vi "reward_behavior_michelle_visjitter_conswinAdapt_enticefx_TSLog_VF_fortraining_lightdetection.vi"() -> ()   [LabVIEW 2019]
doc: "The myRIO Project template acquires acceleration data from the onboard accelerometer and displays the changes of acceleration values in a waveform chart."
uses:
  <vilib>/Analysis/Matrix/Datatypes/RealMatrix.ctl
  <vilib>/myRIO/Instrument Drivers/Onboard IO/DIO/typedefs/DIO Reference.ctl
  <vilib>/myRIO/Common/Instrument Driver Framework/Utilities/typedefs/myRIO Generic Hardware Reference.ctl
  <vilib>/myRIO/Common/Instrument Driver Framework/Utilities/typedefs/Hardware Version Enum.ctl
  <vilib>/myRIO/Common/Instrument Driver Framework/Utilities/typedefs/myRIO v1.0 Reference.ctl
  <vilib>/myRIO/Common/Instrument Driver Framework/Utilities/typedefs/Generic FPGA Reference.ctl
  <vilib>/myRIO/Common/Instrument Driver Framework/myRIO v1.0/DIO/typedefs/DIO Channels List.ctl
  <vilib>/myRIO/Common/Instrument Driver Framework/myRIO v1.0/DIO/typedefs/DIO Channels Enum.ctl
  <vilib>/userdefined/High Color/nirio_resource_hc.ctl
  <vilib>/myRIO/Common/Instrument Driver Framework/myRIO v1.0/Encoder/typedefs/Encoder Signal Mode.ctl
  <vilib>/myRIO/Instrument Drivers/Onboard IO/Encoder/typedefs/Encoder Reference.ctl
  <vilib>/myRIO/Common/Instrument Driver Framework/myRIO v1.0/Encoder/typedefs/Encoder Channels Enum.ctl
  <vilib>/myRIO/Common/Instrument Driver Framework/myRIO v1.0/Encoder/typedefs/Encoder Configuration v1.0.ctl
  <vilib>/myRIO/Instrument Drivers/Onboard IO/AI/typedefs/AI Reference.ctl
  <vilib>/myRIO/Common/Instrument Driver Framework/myRIO v1.0/AI/typedefs/AI Channels List.ctl
  <vilib>/myRIO/Common/Instrument Driver Framework/myRIO v1.0/AI/typedefs/AI Channels Enum.ctl
  <vilib>/myRIO/Common/Instrument Driver Framework/Utilities/typedefs/Analog Scaling Constants List.ctl
  <vilib>/myRIO/Common/Instrument Driver Framework/Utilities/typedefs/Analog Scaling Constants.ctl
  <vilib>/myRIO/Common/Instrument Driver Framework/Utilities/vis/Is FPGA Ref Available.vi
  <vilib>/myRIO/Common/Instrument Driver Framework/myRIO v1.0/DIO/vis/myRIO v1.1 Open DIO.vi
  <vilib>/myRIO/Instrument Drivers/Onboard IO/DIO/vis/Write.vi
  <vilib>/myRIO/Common/Instrument Driver Framework/myRIO v1.0/Encoder/vis/myRIO v1.1 Open Encoder.vi
  <vilib>/myRIO/Instrument Drivers/Onboard IO/Encoder/vis/Read.vi
  <vilib>/myRIO/Common/Instrument Driver Framework/myRIO v1.0/AI/vis/myRIO v1.1 Open AI.vi
  <vilib>/myRIO/Instrument Drivers/Onboard IO/AI/vis/Read.vi
  <vilib>/myRIO/Instrument Drivers/Onboard IO/DIO/vis/Read.vi
  <vilib>/myRIO/Common/Instrument Driver Framework/Utilities/vis/Validate Channels.vi
  <vilib>/myRIO/Common/Instrument Driver Framework/myRIO v1.0/DIO/vis/myRIO v1.0 Reserve DIO.vi
  <vilib>/myRIO/Common/Instrument Driver Framework/myRIO v1.0/Encoder/vis/myRIO v1.0 Reserve Encoder.vi
  <vilib>/myRIO/Common/Instrument Driver Framework/myRIO v1.0/AI/vis/myRIO v1.0 Reserve AI.vi
  <vilib>/myRIO/Common/Instrument Driver Framework/myRIO v1.0/Resource Manager/vis/myRIO v1.0 Reserve Channel List.vi
  <vilib>/myRIO/Common/Instrument Driver Framework/myRIO v1.0/DIO/vis/myRIO v1.0 Build MUX Configuration DIO.vi
  <vilib>/myRIO/Common/Instrument Driver Framework/myRIO v1.0/Encoder/vis/myRIO v1.0 Build MUX Configuration Encoder.vi
  <vilib>/myRIO/Common/Instrument Driver Framework/myRIO v1.0/AI/vis/myRIO v1.0 Build MUX Configuration AI.vi
  <vilib>/myRIO/Common/Instrument Driver Framework/myRIO v1.0/Resource Manager/vis/myRIO v1.0 Reserve Channel.vi
  <vilib>/myRIO/Common/Instrument Driver Framework/myRIO v1.0/Resource Manager/vis/myRIO v1.0 Unreserve Channel.vi
  <vilib>/myRIO/Common/Instrument Driver Framework/myRIO v1.0/Resource Manager/vis/myRIO v1.0 Create Configuration List.vi
  <vilib>/myRIO/Common/Instrument Driver Framework/myRIO v1.0/Resource Manager/vis/myRIO v1.0 Build Mutex Name.vi
  <vilib>/Utility/VariantDataType/GetNumericInfo.vi
  <vilib>/Utility/error.llb/Error Cluster From Error Code.vi
  <vilib>/myRIO/Common/Instrument Driver Framework/myRIO v1.0/myRIO v1.1 Open.vi
  <vilib>/myRIO/Common/Instrument Driver Framework/Utilities/vis/IO Manager.vi
  <vilib>/myRIO/Common/Instrument Driver Framework/Utilities/vis/Configuration Manager.vi
  <vilib>/myRIO/Common/Instrument Driver Framework/myRIO v1.0/Resource Manager/vis/myRIO v1.0 Configure IO.vi
  <vilib>/myRIO/Common/Instrument Driver Framework/myRIO v1.0/myRIO v1.0 Close.vi
  <vilib>/myRIO/Common/Instrument Driver Framework/myRIO v1.0/Encoder/vis/myRIO v1.0 Configure Encoder.vi
  <vilib>/myRIO/Common/Instrument Driver Framework/myRIO v1.0/Encoder/vis/myRIO v1.0 Read Encoder.vi
  <vilib>/myRIO/Common/Instrument Driver Framework/myRIO v1.0/DIO/vis/myRIO v1.0 Write DIO.vi
  <vilib>/myRIO/Common/Instrument Driver Framework/myRIO v1.0/DIO/vis/myRIO v1.0 Read DIO.vi
  <vilib>/myRIO/Common/Instrument Driver Framework/myRIO v1.0/AI/vis/myRIO v1.0 Get Scaling Constants AI.vi
  <vilib>/myRIO/Common/Instrument Driver Framework/myRIO v1.0/AI/vis/myRIO v1.0 Read AI.vi
  <vilib>/myRIO/Express VI/Onboard IO/Encoder/Encoder Express VI.xnode
  <vilib>/myRIO/Instrument Drivers/Onboard IO/Encoder/vis/myRIO Encoder Open.xnode
  <vilib>/myRIO/Common/Instrument Driver Framework/myRIO v1.0/Encoder/typedefs/Encoder Count Direction Enum.ctl
  <vilib>/myRIO/Express VI/Onboard IO/DO/DO Express VI.xnode
  <vilib>/myRIO/Instrument Drivers/Onboard IO/DIO/vis/myRIO DIO Open.xnode
  <vilib>/myRIO/Express VI/Onboard IO/DI/DI Express VI.xnode
  <vilib>/myRIO/Express VI/Onboard IO/AI/AI Express VI.xnode
  <vilib>/myRIO/Instrument Drivers/Onboard IO/AI/vis/myRIO AI Open.xnode
  <vilib>/myRIO/Instrument Drivers/Onboard IO/Encoder/Encoder.lvlib
  <vilib>/myRIO/Instrument Drivers/Onboard IO/DIO/DIO.lvlib
  <vilib>/myRIO/Instrument Drivers/Onboard IO/AI/AI.lvlib
  <vilib>/Analysis/Matrix/NI_Matrix.lvlib
panel:
  out "LightDeriv":dbl
  out "LightOn":bool=TRUE
  out "Light":dbl
  out "Lightplot":dbl[](graph)
  out "LightArray":dbl[](array[numeric])
  out "AutoEnticeLimit":i32=1000
  out "GetVidFrame":i32
  out "VidTS":dbl[][](array[numeric])
  out "VidFrameClock":i32
  out "EntTS":dbl[][](array[numeric])
  out "TimeLag":dbl
  out "Lag2":dbl
  out "TestTime":dbl
  out "RewTS":dbl[][](array[numeric])
  out "ConsTS":dbl[][](array[numeric])
  out "LickTS":dbl[][](array[numeric])
  out "ContrastChoice":dbl
  out "Its":i32
  out "BurstCriteria":dbl
  out "LickBurst 2":bool
  out "LickBurst":bool
  out "Enticements":i32
  in  "Entice":bool
  out "Misses":i32
  out "GoAhead":bool
  out "TimeOutDuration":i32
  out "ActiveTime":dbl
  out "ConsumptionGo":bool=TRUE
  out "Consumption_Period":i32
  out "Watch_Display":bool=TRUE
  in  "Give reward":bool
  out "Timings":dbl[](array[numeric])
  out "ISI":dbl
  out "ISI start time":dbl
  out "Time_out":bool=TRUE
  out "Time since lick":dbl
  out "Time of last lick":dbl
  out "Rewarded trials":dbl[](array[numeric])
  out "Rewards":u16
  out "Active Trial":bool
  out "Array temp2":T1
  out "Stimuli Loaded":bool
  out "Stim_ID":dbl[](array[numeric])
  out "Reward_mat":dbl[](array[numeric])
  out "Reward":bool=TRUE
  out "Frame clock":i32
  out "Licks":u32
  out "Lick":bool
  out "Time":dbl
  out "Stop":bool
  in  "Frames to collect":u32
  out "Overflow?":bool
  out "Counter Value":i32
  out "Velocity":dbl
  out "Velocity Plot":dbl[](graph)
  out "Velocity array":dbl[](array[numeric])
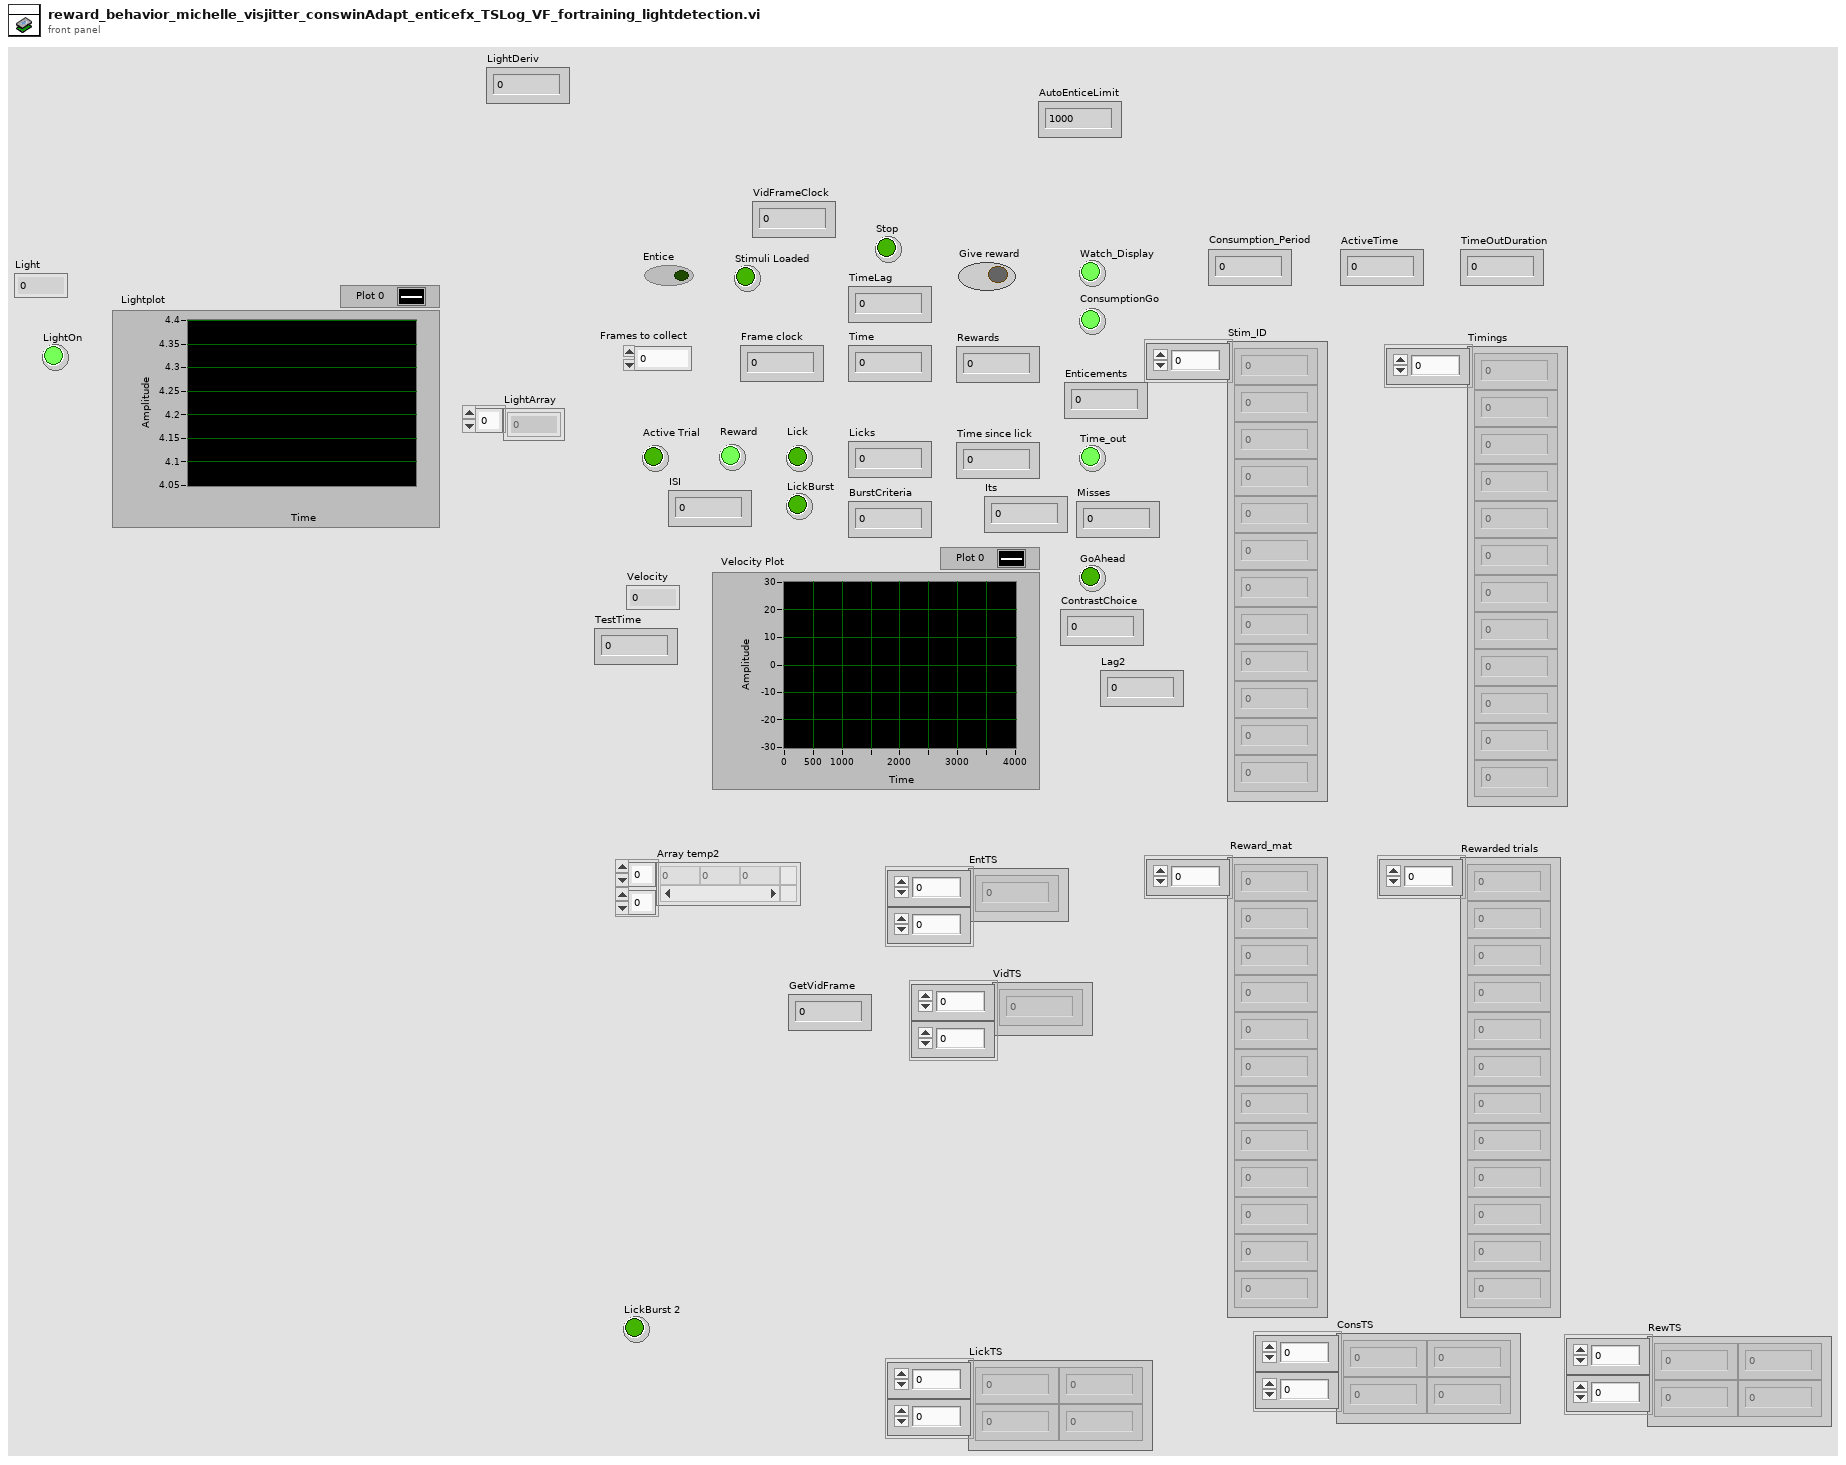
[diagram p1: front panel]
types:
  T1 = typedef "NI_Matrix.lvlib/RealMatrix.ctl" = dbl[][]
  T2 = typedef "DIO.lvlib/DIO Reference.ctl" = cluster{"myRIO Reference":T3, "DIO Channels List":T7}
  T3 = typedef "myRIO Generic Hardware Reference.ctl" = cluster{"myRIO Model":T4, "myRIO Hardware Reference":T5}
  T4 = typedef "Hardware Version Enum.ctl" = enum16{"Unknown", "myRIO-1900", "myRIO-1950", "roboRIO", "NI ELVIS RIO CM", "ELVIS III"}
  T5 = typedef "myRIO v1.0 Reference.ctl" = cluster{"Generic FPGA Reference":T6, "Allow multiple opens":bool}
  T6 = typedef "Generic FPGA Reference.ctl" = refnum<k20>
  T7 = typedef "DIO Channels List.ctl" = T8[]
  T8 = typedef "DIO Channels Enum.ctl" = enum16{"Not Connected", "C/DIO0", "C/DIO1", "C/DIO2", "C/DIO3", "C/DIO4", "C/DIO5", "C/DIO6", "C/DIO7", "A/DIO0", "A/DIO1", "A/DIO2", "A/DIO3", "A/DIO4", "A/DIO5", "A/DIO6", "A/DIO7", "A/DIO8", "A/DIO9", "A/DIO10", "A/DIO11", "A/DIO12", "A/DIO13", "A/DIO14", "A/DIO15", "A/DIO16", "A/DIO17", "A/DIO18", "A/DIO19", "B/DIO0", "B/DIO1", "B/DIO2", "B/DIO3", "B/DIO4", "B/DIO5", "B/DIO6", "B/DIO7", "B/DIO8", "B/DIO9", "B/DIO10", "B/DIO11", "B/DIO12", "B/DIO13", "B/DIO14", "B/DIO15", "B/DIO16", "B/DIO17", "B/DIO18", "B/DIO19", "LED0", "LED1", "LED2", "LED3", "Button0", "DIO/DIO0", "DIO/DIO1", "DIO/DIO2", "DIO/DIO3", "DIO/DIO4", "DIO/DIO5", "DIO/DIO6", "DIO/DIO7", "DIO/DIO8", "DIO/DIO9", "SPI/CS0", "SPI/CS1", "SPI/CS2", "SPI/CS3", "LED RADIO (Green)", "LED RADIO (Red)", "LED COMM (Green)", "LED COMM (Red)", "LED MODE (Green)", "LED MODE (Red)"}
  T9 = typedef "nirio_resource_hc.ctl" = tag
  T10 = typedef "Encoder.lvlib/Encoder Reference.ctl" = cluster{"myRIO Reference":T3, "Encoder Channels Enum":T11}
  T11 = typedef "Encoder Channels Enum.ctl" = enum16{"Not Connected", "C/ENC0", "C/ENC1", "A/ENC", "A/ENC0", "A/ENC1", "A/ENC2", "A/ENC3", "A/ENC4", "A/ENC5", "A/ENC6", "A/ENC7", "A/ENC8", "A/ENC9", "B/ENC", "B/ENC0", "B/ENC1", "B/ENC2", "B/ENC3", "B/ENC4", "B/ENC5", "B/ENC6", "B/ENC7", "B/ENC8", "B/ENC9", "DIO/ENC0", "DIO/ENC1", "DIO/ENC2", "DIO/ENC3", "DIO/ENC4"}
  T12 = typedef "Encoder Signal Mode.ctl" = enum16{"Quadrature phase signal", "Step and direction signal"}
  T13 = typedef "AI.lvlib/AI Reference.ctl" = cluster{"myRIO Reference":T3, "AI Channels List":T14, "AI Scaling Constants List":T16}
  T14 = typedef "AI Channels List.ctl" = T15[]
  T15 = typedef "AI Channels Enum.ctl" = enum16{"Not Connected", "AudioIn/Left", "AudioIn/Right", "C/AI0", "C/AI1", "A/AI0", "A/AI1", "A/AI2", "A/AI3", "A/AI4", "A/AI5", "A/AI6", "A/AI7", "B/AI0", "B/AI1", "B/AI2", "B/AI3", "B/AI4", "B/AI5", "B/AI6", "B/AI7", "AI/AI0", "AI/AI1", "AI/AI2", "AI/AI3", "A/AI0 (DIFF)", "A/AI1 (DIFF)", "A/AI2 (DIFF)", "A/AI3 (DIFF)", "B/AI0 (DIFF)", "B/AI1 (DIFF)", "B/AI2 (DIFF)", "B/AI3 (DIFF)"}
  T16 = typedef "Analog Scaling Constants List.ctl" = T17[]
  T17 = typedef "Analog Scaling Constants.ctl" = cluster{"LSB Weight (Volts)":dbl, "Offset (Volts)":dbl, "Signed?":bool}
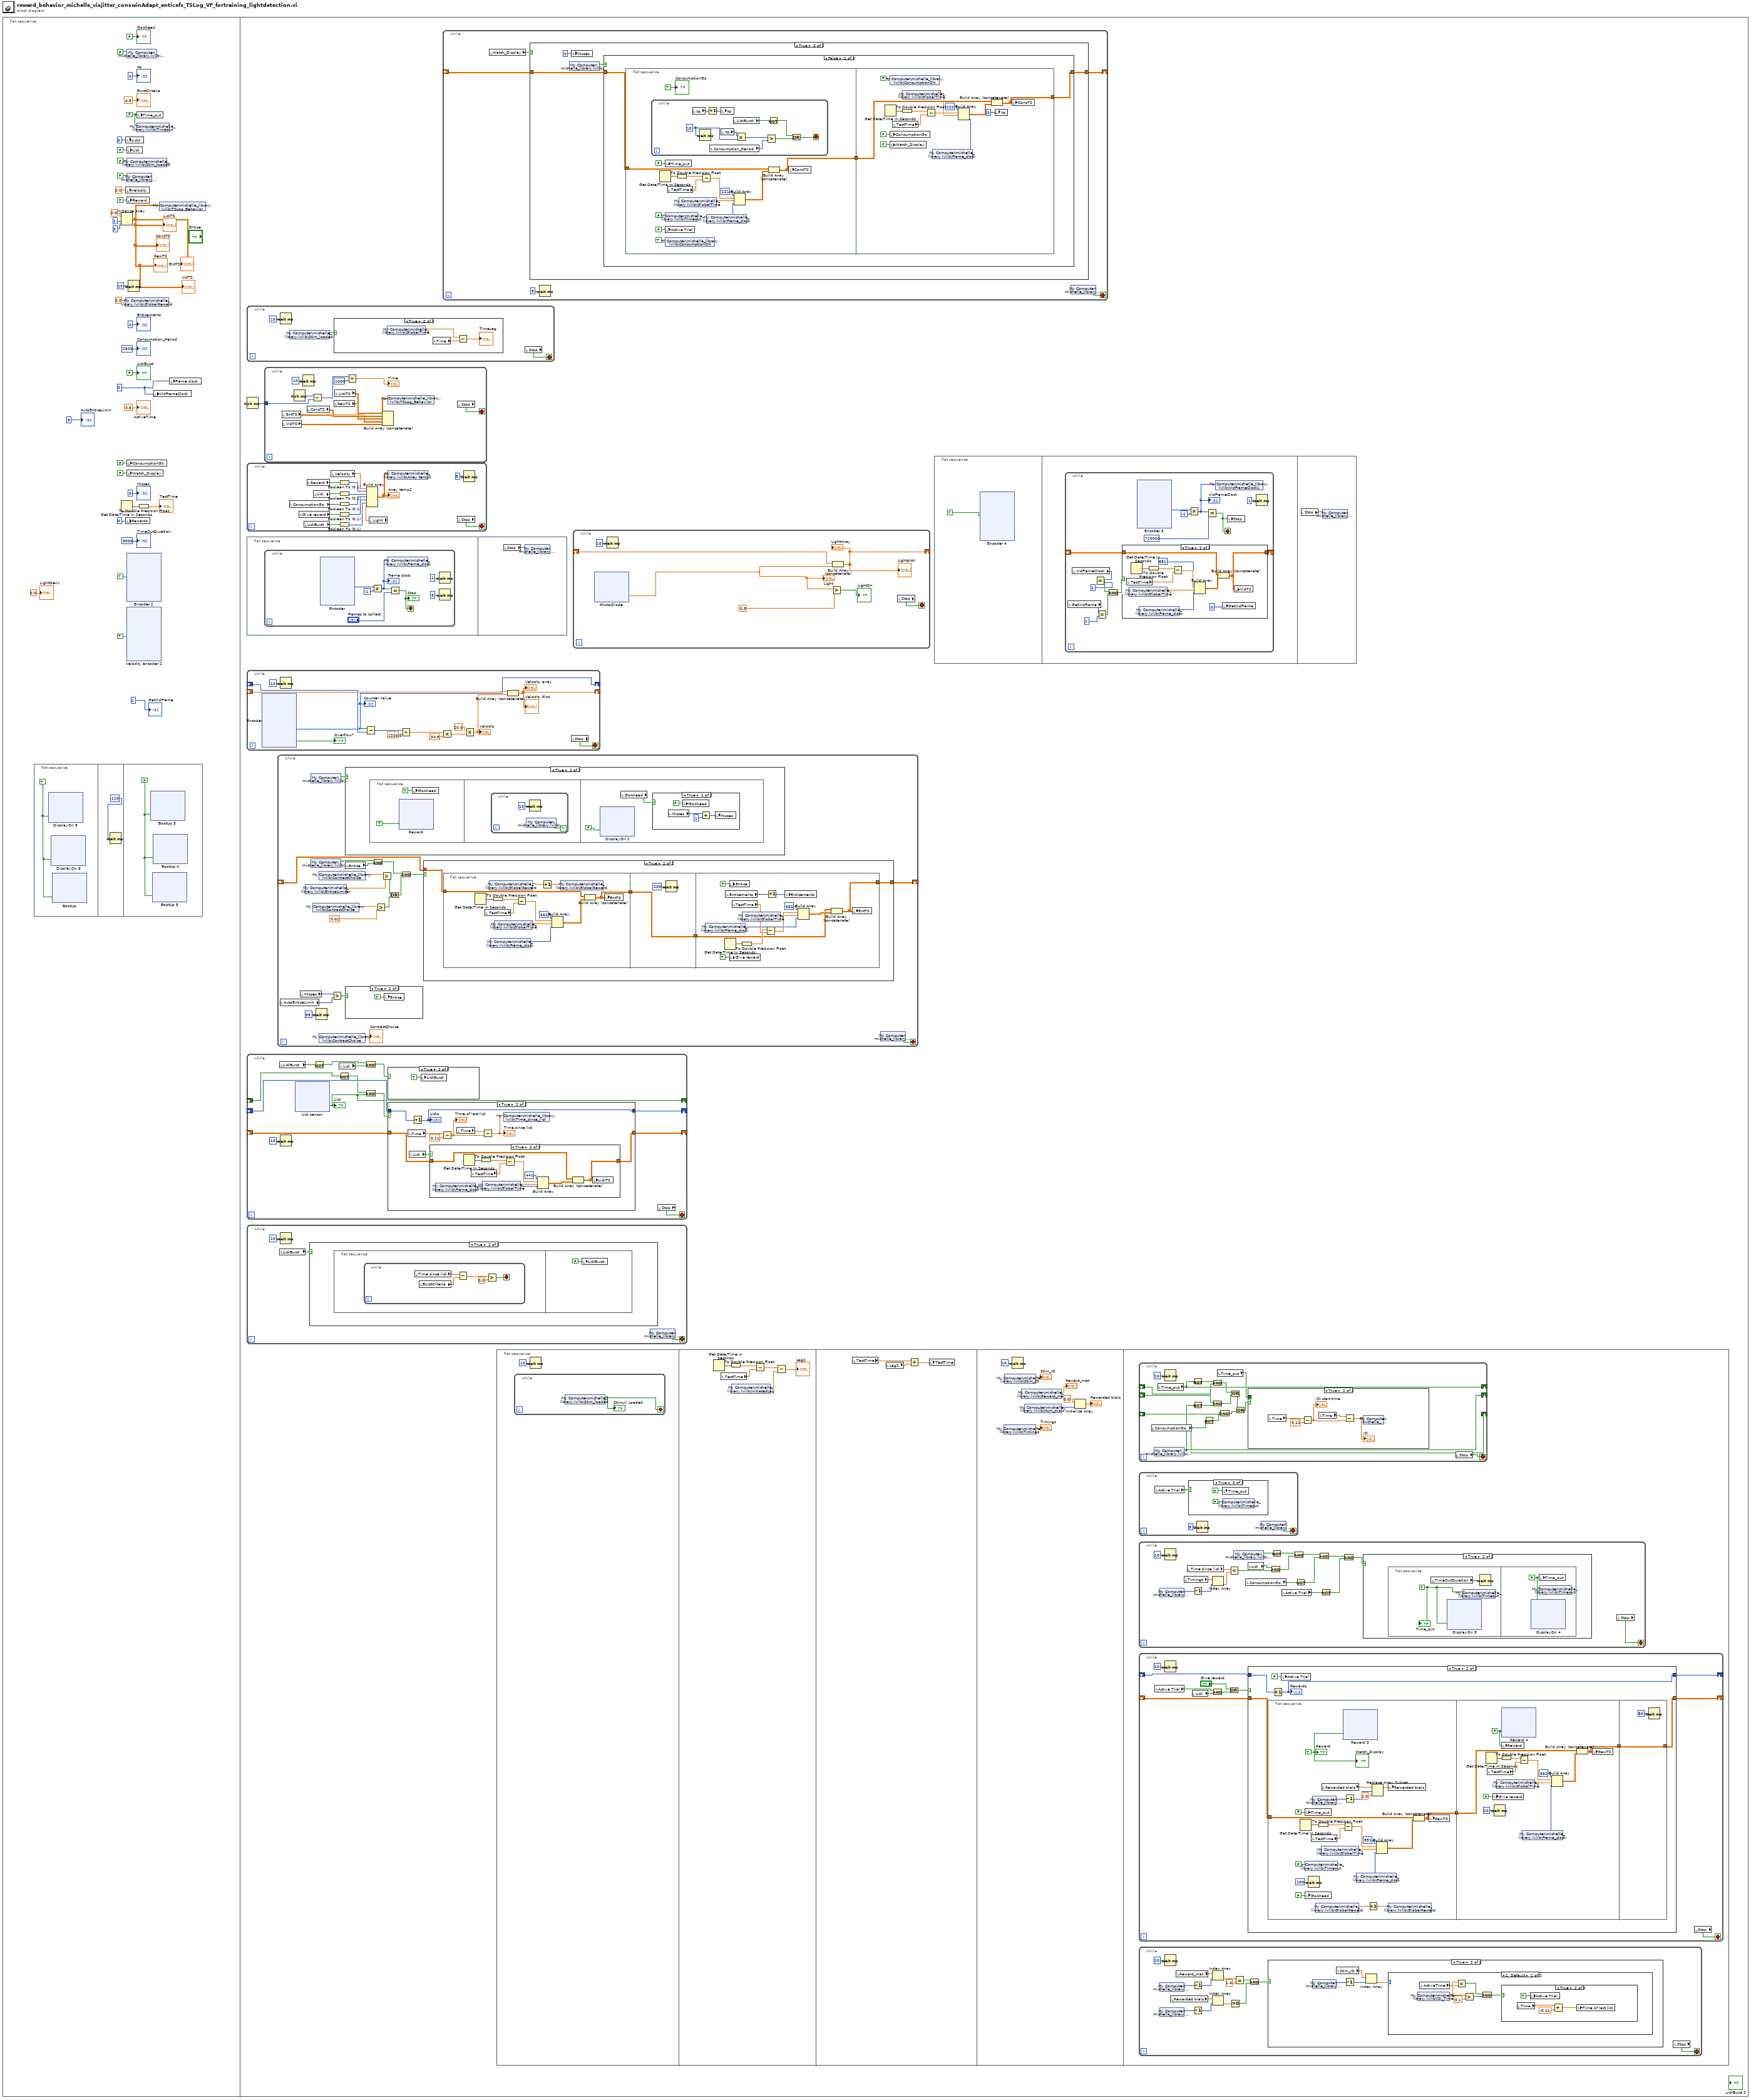
[diagram p0: block diagram]
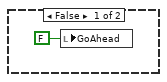
[diagram p7: hidden frame]
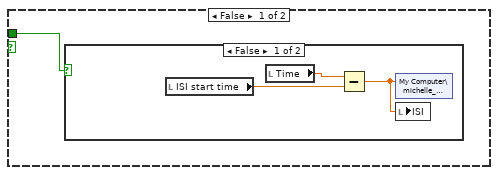
[diagram p13: hidden frame]
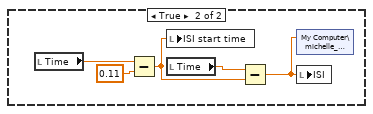
[diagram p14: hidden frame]
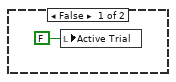
[diagram p15: hidden frame]
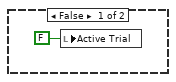
[diagram p16: hidden frame]
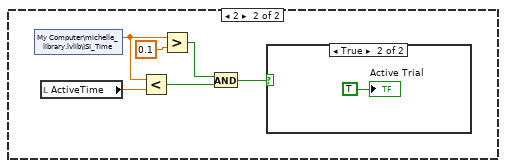
[diagram p17: hidden frame]
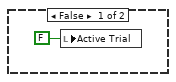
[diagram p18: hidden frame]
diagram:
  n1 = flat-sequence {
    frame #0 {
      w23 = FALSE ("Time_out")
      w5 = u32 0 ("Frames")
      n2 = flat-sequence {
        frame #0 {
          w35 = TRUE
          n3 = xnode "DisplayOn 5"("C/DIO2 (DIO2)"=w35) -> ()  [unwired: 1 in, 1 out]
          n4 = xnode "DisplayOn 6"("C/DIO1 (DIO1)"=w35) -> ()  [unwired: 1 in, 1 out]
          n5 = xnode "BootUp"("C/DIO3 (DIO3)"=w35) -> ()  [unwired: 1 in, 1 out]
        }
        frame #1 {
          n6 = Wait (ms)(milliseconds to wait=210) -> ()  [unwired: 1 out]
        }
        frame #2 {
          w142 = FALSE
          n7 = xnode "BootUp 3"("C/DIO2 (DIO2)"=w142) -> ()  [unwired: 1 in, 1 out]
          n8 = xnode "BootUp 5"("C/DIO3 (DIO3)"=w142) -> ()  [unwired: 1 in, 1 out]
          n9 = xnode "BootUp 4"("C/DIO1 (DIO1)"=w142) -> ()  [unwired: 1 in, 1 out]
        }
      }
      n10 = Get Date/Time In Seconds() -> (seconds since 1Jan1904=w7:timestamp)
      n11 = Initialize Array(0.0, 1, 3) -> (w4:dbl[][])
      "LickTS" <- w4
      "ConsTS" <- w4
      "RewTS" <- w4
      "EntTS" <- w4
      "VidTS" <- w4
      n12 = local write "Licks"(u32 0 ("Licks")) -> ()
      n13 = local write "Velocity"(0.0 ("Velocity")) -> ()
      n14 = shared-variable "My Computer\\michelle_library.lvlib\\GlobalReward"(0.0) -> ()  [unwired: 1 in, 1 out]
      n15 = local write "Rewards"(u16 0 ("Rewards")) -> ()
      n16 = shared-variable "My Computer\\michelle_library.lvlib\\Display"(FALSE ("Display")) -> ()  [unwired: 1 in, 1 out]
      n17 = local write "Lick"(FALSE ("Lick")) -> ()
      n18 = shared-variable "My Computer\\michelle_library.lvlib\\Stim_loaded"(FALSE ("Stim_loaded")) -> ()  [unwired: 1 in, 1 out]
      n19 = shared-variable "My Computer\\michelle_library.lvlib\\Stop"(FALSE ("Stop")) -> ()  [unwired: 1 in, 1 out]
      n20 = local write "Reward"(FALSE ("Give reward")) -> ()
      n21 = local write "ConsumptionGo"(FALSE ("ConsumptionGo")) -> ()
      n22 = local write "Watch_Display"(FALSE ("Watch_Display")) -> ()
      n23 = xnode "Encoder 2"("Reset Counter"=TRUE) -> ()  [unwired: 1 in, 4 out]
      n24 = xnode "Velocity encoder 2"("Reset Counter"=TRUE) -> ()  [unwired: 1 in, 4 out]
      n25 = Wait (ms)(milliseconds to wait=u32 10) -> ()  [unwired: 1 out]
      n26 = local write "Time_out"(w23) -> ()
      n27 = shared-variable "My Computer\\michelle_library.lvlib\\Timeout"(w23) -> ()  [unwired: 1 in, 1 out]
      n28 = To Double Precision Float(number=w7) -> (double precision float=→"TestTime":dbl)
      n29 = local write "VidFrameClock"(w5) -> ()
      n30 = shared-variable "My Computer\\michelle_library.lvlib\\TSLog_Behavior"(w4) -> ()  [unwired: 1 in, 1 out]
      n31 = local write "Frame clock"(w5) -> ()
      "Consumption_Period" <- 2500
      "ActiveTime" <- 0.6
      "TimeOutDuration" <- 3000
      "GoAhead" <- FALSE
      "Misses" <- 0
      "Enticements" <- 0
      "LickBurst" <- FALSE
      "BurstCriteria" <- 0.5
      "Its" <- 0
      "GetVidFrame" <- 1
      "AutoEnticeLimit" <- 5
      "LightDeriv" <- 0.0
    }
    frame #1 {
      n32 = while {
        stop <- w507 stop-if-true
        n33 = Wait (ms)(milliseconds to wait=u32 10) -> ()  [unwired: 1 out]
        n34 = shared-variable "My Computer\\michelle_library.lvlib\\Stim_loaded"() -> (w508:bool)  [unwired: 1 in, 1 out]
        n35 = case shown="True" w508 {
          frame False {
          }
          frame True {
            n36 = shared-variable "My Computer\\michelle_library.lvlib\\GlobalTime"() -> (w509:dbl)  [unwired: 1 in, 1 out]
            n37 = local read "Time"() -> (w510:dbl)
            n38 = Subtract(x=w509, y=w510) -> (x-y=→"TimeLag":dbl)
          }
        }
        n39 = local read "Stop"() -> (w507:bool)
      }
      n40 = Tick Count (ms)() -> (millisecond timer value=w340:u32)
      n41 = while {
        stop <- w717 stop-if-true
        n42 = local read "ConsumptionGo"() -> (w715:bool)
        n43 = local read "Give reward"() -> (w714:bool)
        n44 = local read "LickBurst"() -> (w711:bool)
        n45 = local read "Reward"() -> (w722:bool)
        n46 = local read "Lick"() -> (w723:bool)
        n47 = local read "Velocity"() -> (w721:dbl)
        n48 = Boolean To (0,1)(Boolean=w722) -> (0, 1=w720:i16)
        n49 = Boolean To (0,1)(Boolean=w723) -> (0, 1=w719:i16)
        n50 = Boolean To (0,1)(Boolean=w715) -> (0, 1=w713:i16)
        n51 = Boolean To (0,1)(Boolean=w714) -> (0, 1=w712:i16)
        n52 = Boolean To (0,1)(Boolean=w711) -> (0, 1=w710:i16)
        n53 = local read "Light"() -> (w709:dbl)
        n54 = Build Array(w721, w720, w719, w713, w712, w710, w709) -> (w716:T1)
        "Array temp2" <- w716
        n55 = shared-variable "My Computer\\michelle_library.lvlib\\Array temp2"(w716) -> ()  [unwired: 1 in, 1 out]
        n56 = local read "Stop"() -> (w717:bool)
        n57 = Wait (ms)(milliseconds to wait=u32 5) -> ()  [unwired: 1 out]
      }
      n58 = flat-sequence {
        frame #0 {
          n59 = while {
            stop <- w1036 stop-if-true
            n60 = xnode "Encoder"() -> ("Counter Value"=w1040:i32)  [unwired: 2 in, 3 out]
            n61 = Multiply(x=w1040, y=-1) -> (x*y=w1035:i32)
            "Frame clock" <- w1035
            n62 = shared-variable "My Computer\\michelle_library.lvlib\\Frame_clock"(w1035) -> ()  [unwired: 1 in, 1 out]
            n63 = Equal?(x=w1035, y="Frames to collect") -> (x = y?=w1036:bool)
            "Stop" <- w1036
            n64 = Wait (ms)(milliseconds to wait=u32 1) -> ()  [unwired: 1 out]
            n65 = Wait (ms)(milliseconds to wait=u32 5) -> ()  [unwired: 1 out]
          }
        }
        frame #1 {
          n66 = local read "Stop"() -> (w1088:bool)
          n67 = shared-variable "My Computer\\michelle_library.lvlib\\Stop"(w1088) -> ()  [unwired: 1 in, 1 out]
        }
      }
      n68 = while {
        shift-right: [w1175] -> _
        shift-left: _ -> [w1176]
        shift-right: [w1167] -> _
        shift-left: _ -> [w1166]
        stop <- w1165 stop-if-true
        n69 = xnode "Encoder"() -> ("Counter Value"=w1175:i32, "Overflow?"=→"Overflow?":bool)  [unwired: 2 in, 2 out]
        "Counter Value" <- w1175
        n70 = Wait (ms)(milliseconds to wait=u32 10) -> ()  [unwired: 1 out]
        n71 = Subtract(x=w1175, y=w1176) -> (x-y=w1168:i32)
        n72 = Divide(x=w1168, y=1200.0 ("600")) -> (x/y=w1173:dbl)
        n73 = Multiply(x=w1173, y=34.5) -> (x*y=w1171:dbl)
        n74 = Multiply(x=20.0, y=w1171) -> (x*y=w1169:dbl)
        "Velocity" <- w1169
        n75 = Build Array (concatenate)(w1166, w1169) -> (w1167:dbl[])
        "Velocity Plot" <- w1167
        "Velocity array" <- w1167
        n76 = local read "Stop"() -> (w1165:bool)
      }
      n77 = while {
        shift-right: [w1101] -> _
        shift-left: _ -> [w1100]
        shift-right: [w1095] -> _
        shift-left: _ -> [w1098]
        shift-right: [w1089] -> _
        shift-left: _ -> [w1090]
        stop <- w1099 stop-if-true
        n78 = local read "LickBurst"() -> (w1092:bool)
        n79 = Wait (ms)(milliseconds to wait=u32 10) -> ()  [unwired: 1 out]
        n80 = xnode "Lick sensor"() -> ("C/DIO1 (DIO1)"=w1095:bool)  [unwired: 1 in, 1 out]
        "Lick" <- w1095
        n81 = Not(x=w1092) -> (.not. x?=w1091:bool)
        n82 = Not(x=w1098) -> (.not. x?=w1097:bool)
        n83 = local read "Lick"() -> (w1093:bool)
        n84 = And(x=w1091, y=w1093) -> (x .and. y?=w1094:bool)
        n85 = And(x=w1097, y=w1095) -> (x .and. y?=w1096:bool)
        n86 = case shown="True" w1094 {
          frame False {
          }
          frame True {
            n87 = local write "LickBurst"(TRUE) -> ()
          }
        }
        n88 = case shown="True" w1096 {
          tunnel: [w1108 w1118] -> w1101
          tunnel: w1100 -> [w1108 w1117]
          tunnel: w1090 -> [w1104 w1109]
          tunnel: [w1104 w1111] -> w1089
          frame False {
            n89 = local read "Time of last lick"() -> (w1106:dbl)
            n90 = local read "Time"() -> (w1107:dbl)
            n91 = Subtract(x=w1107, y=w1106) -> (x-y=w1105:dbl)
            n92 = shared-variable "My Computer\\michelle_library.lvlib\\Time_since_lick"(w1105) -> ()  [unwired: 1 in, 1 out]
            n93 = local write "Time since lick"(w1105) -> ()
          }
          frame True {
            n94 = local read "Time"() -> (w1114:dbl)
            n95 = local read "Lick"() -> (w1110:bool)
            n96 = Increment(x=w1117) -> (x+1=w1118:u32)
            "Licks" <- w1118
            n97 = case shown="True" w1110 {
              tunnel: w1109 -> [w1119 w1125]
              tunnel: [w1119 w1124] -> w1111
              frame False {
              }
              frame True {
                n98 = shared-variable "My Computer\\michelle_library.lvlib\\Frame_clock"() -> (w1120:u32)  [unwired: 1 in, 1 out]
                n99 = Get Date/Time In Seconds() -> (seconds since 1Jan1904=w1127:timestamp)
                n100 = local read "TestTime"() -> (w1122:dbl)
                n101 = To Double Precision Float(number=w1127) -> (double precision float=w1123:dbl)
                n102 = shared-variable "My Computer\\michelle_library.lvlib\\GlobalTime"() -> (w1121:dbl)  [unwired: 1 in, 1 out]
                n103 = Subtract(x=w1123, y=w1122) -> (x-y=w1128:dbl)
                n104 = Build Array(441, w1128, w1121, w1120) -> (w1129:T1)
                n105 = Build Array (concatenate) ("Build Matrix")(w1125, w1129) -> (w1124:T1)
                n106 = local write "LickTS"(w1124) -> ()
              }
            }
            n107 = Subtract(x=w1114, y=0.11) -> (x-y=w1112:dbl)
            "Time of last lick" <- w1112
            n108 = local read "Time"() -> (w1116:dbl)
            n109 = Subtract(x=w1116, y=w1112) -> (x-y=w1115:dbl)
            "Time since lick" <- w1115
            n110 = shared-variable "My Computer\\michelle_library.lvlib\\Time_since_lick"(w1115) -> ()  [unwired: 1 in, 1 out]
          }
        }
        n111 = local read "Stop"() -> (w1099:bool)
      }
      n112 = while {
        stop <- w514 stop-if-true
        n113 = local read "LickBurst"() -> (w512:bool)
        n114 = Wait (ms)(milliseconds to wait=u32 10) -> ()  [unwired: 1 out]
        n115 = case shown="True" w512 {
          frame False {
          }
          frame True {
            n116 = flat-sequence {
              frame #0 {
                n117 = while {
                  stop <- w517 stop-if-true
                  n118 = local read "Time since lick"() -> (w518:dbl)
                  n119 = local read "BurstCriteria"() -> (w519:dbl)
                  n120 = Subtract(x=w518, y=w519) -> (x-y=w515:dbl)
                  n121 = Greater?(x=w515, y=0.0) -> (0:w517:bool)
                }
              }
              frame #1 {
                n122 = local write "LickBurst"(FALSE) -> ()
              }
            }
          }
        }
        n123 = shared-variable "My Computer\\michelle_library.lvlib\\Stop"() -> (w514:bool)  [unwired: 1 in, 1 out]
      }
      n124 = while {
        tunnel: w340 -> [w1236]
        stop <- w1234 stop-if-true
        n125 = local read "EntTS"() -> (w1226:dbl[][])
        n126 = local read "VidTS"() -> (w1225:dbl[][])
        n127 = Tick Count (ms)() -> (millisecond timer value=w1237:u32)
        n128 = Wait (ms)(milliseconds to wait=u32 10) -> ()  [unwired: 1 out]
        n129 = local read "ConsTS"() -> (w1229:dbl[][])
        n130 = Subtract(x=w1237, y=w1236) -> (x-y=w1233:u32)
        n131 = local read "RewTS"() -> (w1228:dbl[][])
        n132 = local read "LickTS"() -> (w1230:dbl[][])
        n133 = Divide(x=w1233, y=u32 1000) -> (x/y=→"Time":dbl)
        n134 = Build Array (concatenate) ("Build Matrix")(w1230, w1229, w1228, w1226, w1225) -> (w1227:T1)
        n135 = shared-variable "My Computer\\michelle_library.lvlib\\TSLog_Behavior"(w1227) -> ()  [unwired: 1 in, 1 out]
        n136 = local read "Stop"() -> (w1234:bool)
      }
      n137 = while {
        shift-right: [w529] -> _
        shift-left: _ -> [w530]
        stop <- w540 stop-if-true
        n138 = local read "AutoEnticeLimit"() -> (w521:i32)
        n139 = local read "Misses"() -> (w522:i32)
        n140 = shared-variable "My Computer\\michelle_library.lvlib\\EnticeLimiter"() -> (w528:dbl)  [unwired: 1 in, 1 out]
        n141 = shared-variable "My Computer\\michelle_library.lvlib\\Display"() -> (w539:bool)  [unwired: 1 in, 1 out]
        n142 = shared-variable "My Computer\\michelle_library.lvlib\\Display"() -> (w537:bool)  [unwired: 1 in, 1 out]
        n143 = shared-variable "My Computer\\michelle_library.lvlib\\ContrastChoice"() -> (w524:dbl)  [unwired: 1 in, 1 out]
        n144 = Wait (ms)(milliseconds to wait=35) -> ()  [unwired: 1 out]
        n145 = shared-variable "My Computer\\michelle_library.lvlib\\ContrastChoice"() -> (w533:dbl)  [unwired: 1 in, 1 out]
        n146 = shared-variable "My Computer\\michelle_library.lvlib\\ContrastChoice"() -> (→"ContrastChoice":dbl)  [unwired: 1 in, 1 out]
        n147 = Greater?(x=w522, y=w521) -> (0:w538:bool)
        n148 = case shown="True" w539 {
          frame False {
            n149 = local write "GoAhead"(FALSE) -> ()
          }
          frame True {
            n150 = flat-sequence {
              frame #0 {
                n151 = xnode "Reward"("C/DIO2 (DIO2)"=TRUE) -> ()  [unwired: 1 in, 1 out]
                n152 = local write "GoAhead"(TRUE) -> ()
              }
              frame #1 {
                n153 = while {
                  stop <- w614 continue-if-true
                  n154 = shared-variable "My Computer\\michelle_library.lvlib\\Display"() -> (w614:bool)  [unwired: 1 in, 1 out]
                  n155 = Wait (ms)(milliseconds to wait=10) -> ()  [unwired: 1 out]
                }
              }
              frame #2 {
                n156 = xnode "DisplayOn 2"("C/DIO2 (DIO2)"=FALSE) -> ()  [unwired: 1 in, 1 out]
                n157 = local read "GoAhead"() -> (w616:bool)
                n158 = case shown="True" w616 {
                  frame False {
                  }
                  frame True {
                    n159 = local read "Misses"() -> (w655:i32)
                    n160 = local write "GoAhead"(FALSE) -> ()
                    n161 = Add(x=w655, y=1) -> (x+y=w653:i32)
                    n162 = local write "Misses"(w653) -> ()
                  }
                }
              }
            }
          }
        }
        n163 = local read "Entice"() -> (w536:bool)
        n164 = case shown="True" w538 {
          frame False {
          }
          frame True {
            n165 = local write "Entice"(TRUE) -> ()
          }
        }
        n166 = And(x=w537, y=w536) -> (x .and. y?=w534:bool)
        n167 = Greater?(x=w524, y=0.02) -> (0:w525:bool)
        n168 = Greater?(x=w533, y=w528) -> (0:w526:bool)
        n169 = Or(x=w526, y=w525) -> (x .or. y?=w527:bool)
        n170 = And(x=w534, y=w527) -> (x .and. y?=w532:bool)
        n171 = case shown="True" w532 {
          tunnel: w530 -> [w541 w545]
          tunnel: [w541 w542] -> w529
          frame False {
          }
          frame True {
            n172 = flat-sequence {
              tunnel: w545 -> [w548]
              tunnel: [w547] -> w544
              tunnel: w544 -> [w558]
              tunnel: [w558] -> w543
              tunnel: w543 -> [w562]
              tunnel: [w561] -> w542
              frame #0 {
                n173 = Get Date/Time In Seconds() -> (seconds since 1Jan1904=w555:timestamp)
                n174 = local read "TestTime"() -> (w550:dbl)
                n175 = shared-variable "My Computer\\michelle_library.lvlib\\GlobalReward"() -> (w557:dbl)  [unwired: 1 in, 1 out]
                n176 = shared-variable "My Computer\\michelle_library.lvlib\\Frame_clock"() -> (w546:u32)  [unwired: 1 in, 1 out]
                n177 = To Double Precision Float(number=w555) -> (double precision float=w554:dbl)
                n178 = shared-variable "My Computer\\michelle_library.lvlib\\GlobalTime"() -> (w549:dbl)  [unwired: 1 in, 1 out]
                n179 = Subtract(x=w554, y=w550) -> (x-y=w553:dbl)
                n180 = Increment(x=w557) -> (x+1=w556:dbl)
                n181 = Build Array(661, w553, w549, w546) -> (w552:T1)
                n182 = shared-variable "My Computer\\michelle_library.lvlib\\GlobalReward"(w556) -> ()  [unwired: 1 in, 1 out]
                n183 = Build Array (concatenate) ("Build Matrix")(w548, w552) -> (w547:T1)
                n184 = local write "EntTS"(w547) -> ()
              }
              frame #1 {
                n185 = Wait (ms)(milliseconds to wait=200) -> ()  [unwired: 1 out]
              }
              frame #2 {
                n186 = shared-variable "My Computer\\michelle_library.lvlib\\Frame_clock"() -> (w560:u32)  [unwired: 1 in, 1 out]
                n187 = Get Date/Time In Seconds() -> (seconds since 1Jan1904=w569:timestamp)
                n188 = local read "Enticements"() -> (w571:i32)
                n189 = local write "Entice"(FALSE) -> ()
                n190 = local write "Give reward"(TRUE) -> ()
                n191 = local read "TestTime"() -> (w563:dbl)
                n192 = To Double Precision Float(number=w569) -> (double precision float=w568:dbl)
                n193 = shared-variable "My Computer\\michelle_library.lvlib\\GlobalTime"() -> (w564:dbl)  [unwired: 1 in, 1 out]
                n194 = Subtract(x=w568, y=w563) -> (x-y=w567:dbl)
                n195 = Increment(x=w571) -> (x+1=w570:i32)
                n196 = local write "Enticements"(w570) -> ()
                n197 = Build Array(662, w567, w564, w560) -> (w566:T1)
                n198 = Build Array (concatenate) ("Build Matrix")(w562, w566) -> (w561:T1)
                n199 = local write "EntTS"(w561) -> ()
              }
            }
          }
        }
        n200 = shared-variable "My Computer\\michelle_library.lvlib\\Stop"() -> (w540:bool)  [unwired: 1 in, 1 out]
      }
      n201 = while {
        shift-right: [w656] -> _
        shift-left: _ -> [w657]
        stop <- w660 stop-if-true
        n202 = local read "Watch_Display"() -> (w659:bool)
        n203 = case shown="True" w659 {
          tunnel: w657 -> [w661 w663]
          tunnel: [w661 w662] -> w656
          frame False {
          }
          frame True {
            n204 = shared-variable "My Computer\\michelle_library.lvlib\\Display"() -> (w665:bool)  [unwired: 1 in, 1 out]
            n205 = local write "Misses"(0) -> ()
            n206 = case shown="False" w665 {
              tunnel: w663 -> [w668 w708]
              tunnel: [w666 w708] -> w662
              frame False {
                n207 = flat-sequence {
                  tunnel: w668 -> [w672]
                  tunnel: [w671] -> w667
                  tunnel: w667 -> [w698]
                  tunnel: [w697] -> w666
                  frame #0 {
                    n208 = while {
                      stop <- w687 stop-if-true
                      w688 = 10
                      n209 = local read "Its"() -> (w692:i32)
                      n210 = Wait (ms)(milliseconds to wait=w688) -> ()  [unwired: 1 out]
                      n211 = Increment(x=w692) -> (x+1=w691:i32)
                      n212 = local read "Consumption_Period"() -> (w685:i32)
                      n213 = local write "Its"(w691) -> ()
                      n214 = local read "Its"() -> (w689:i32)
                      n215 = local read "LickBurst"() -> (w693:bool)
                      n216 = Multiply(x=w689, y=w688) -> (x*y=w686:i32)
                      n217 = Greater?(x=w686, y=w685) -> (0:w684:bool)
                      n218 = Not(x=w693) -> (.not. x?=w690:bool)
                      n219 = Or(x=w690, y=w684) -> (x .or. y?=w687:bool)
                    }
                    n220 = Get Date/Time In Seconds() -> (seconds since 1Jan1904=w677:timestamp)
                    n221 = local write "Time_out"(FALSE) -> ()
                    n222 = shared-variable "My Computer\\michelle_library.lvlib\\Timeout"(FALSE) -> ()  [unwired: 1 in, 1 out]
                    n223 = local write "Active Trial"(FALSE) -> ()
                    n224 = shared-variable "My Computer\\michelle_library.lvlib\\ConsumptionON"(TRUE) -> ()  [unwired: 1 in, 1 out]
                    n225 = local read "TestTime"() -> (w674:dbl)
                    n226 = To Double Precision Float(number=w677) -> (double precision float=w675:dbl)
                    n227 = shared-variable "My Computer\\michelle_library.lvlib\\GlobalTime"() -> (w670:dbl)  [unwired: 1 in, 1 out]
                    n228 = Subtract(x=w675, y=w674) -> (x-y=w678:dbl)
                    n229 = shared-variable "My Computer\\michelle_library.lvlib\\Frame_clock"() -> (w669:u32)  [unwired: 1 in, 1 out]
                    n230 = Build Array(221, w678, w670, w669) -> (w673:T1)
                    n231 = Build Array (concatenate) ("Build Matrix")(w672, w673) -> (w671:T1)
                    n232 = local write "ConsTS"(w671) -> ()
                    "ConsumptionGo" <- TRUE
                  }
                  frame #1 {
                    n233 = Get Date/Time In Seconds() -> (seconds since 1Jan1904=w702:timestamp)
                    n234 = shared-variable "My Computer\\michelle_library.lvlib\\ConsumptionON"(FALSE) -> ()  [unwired: 1 in, 1 out]
                    n235 = local write "ConsumptionGo"(FALSE ("ConsumptionGo")) -> ()
                    n236 = local write "Watch_Display"(FALSE ("Watch_Display")) -> ()
                    n237 = local read "TestTime"() -> (w699:dbl)
                    n238 = To Double Precision Float(number=w702) -> (double precision float=w700:dbl)
                    n239 = shared-variable "My Computer\\michelle_library.lvlib\\GlobalTime"() -> (w695:dbl)  [unwired: 1 in, 1 out]
                    n240 = Subtract(x=w700, y=w699) -> (x-y=w703:dbl)
                    n241 = shared-variable "My Computer\\michelle_library.lvlib\\Frame_clock"() -> (w694:u32)  [unwired: 1 in, 1 out]
                    n242 = Build Array(222, w703, w695, w694) -> (w696:T1)
                    n243 = Build Array (concatenate) ("Build Matrix")(w698, w696) -> (w697:T1)
                    n244 = local write "Its"(0) -> ()
                    n245 = local write "ConsTS"(w697) -> ()
                  }
                }
              }
              frame True {
              }
            }
          }
        }
        n246 = Wait (ms)(milliseconds to wait=u32 5) -> ()  [unwired: 1 out]
        n247 = shared-variable "My Computer\\michelle_library.lvlib\\Stop"() -> (w660:bool)  [unwired: 1 in, 1 out]
      }
      n248 = flat-sequence {
        frame #0 {
          n249 = while {
            stop <- w725 stop-if-true
            n250 = shared-variable "My Computer\\michelle_library.lvlib\\Stim_loaded"() -> (w725:bool)  [unwired: 1 in, 1 out]
            "Stimuli Loaded" <- w725
          }
          n251 = Wait (ms)(milliseconds to wait=u32 10) -> ()  [unwired: 1 out]
        }
        frame #1 {
          n252 = Get Date/Time In Seconds() -> (seconds since 1Jan1904=w731:timestamp)
          n253 = local read "TestTime"() -> (w730:dbl)
          n254 = To Double Precision Float(number=w731) -> (double precision float=w729:dbl)
          n255 = shared-variable "My Computer\\michelle_library.lvlib\\InitiatedLag"() -> (w728:dbl)  [unwired: 1 in, 1 out]
          n256 = Subtract(x=w729, y=w730) -> (x-y=w726:dbl)
          n257 = Subtract(x=w726, y=w728) -> (x-y=→"Lag2":dbl)
        }
        frame #2 {
          n258 = local read "TestTime"() -> (w732:dbl)
          n259 = local read "Lag2"() -> (w733:dbl)
          n260 = Add(x=w732, y=w733) -> (x+y=w734:dbl)
          n261 = local write "TestTime"(w734) -> ()
        }
        frame #3 {
          n262 = shared-variable "My Computer\\michelle_library.lvlib\\Timings"() -> (→"Timings":dbl[])  [unwired: 1 in, 1 out]
          n263 = shared-variable "My Computer\\michelle_library.lvlib\\Stim_ID"() -> (→"Stim_ID":dbl[])  [unwired: 1 in, 1 out]
          n264 = Wait (ms)(milliseconds to wait=u32 10) -> ()  [unwired: 1 out]
          n265 = shared-variable "My Computer\\michelle_library.lvlib\\Reward_mat"() -> (→"Reward_mat":dbl[])  [unwired: 1 in, 1 out]
          n266 = shared-variable "My Computer\\michelle_library.lvlib\\Num_trials"() -> (w738:u32)  [unwired: 1 in, 1 out]
          n267 = Initialize Array(0.0 ("element"), w738) -> (→"Rewarded trials":dbl[])
        }
        frame #4 {
          n268 = while {
            shift-right: [w854] -> _
            shift-left: _ -> [w852]
            shift-right: [w850] -> _
            shift-left: _ -> [w849]
            shift-right: [w844] -> _
            shift-left: _ -> [w842]
            stop <- w855 stop-if-true
            n269 = local read "ConsumptionGo"() -> (w844:bool)
            n270 = shared-variable "My Computer\\michelle_library.lvlib\\Display"() -> (w850:bool)  [unwired: 1 in, 1 out]
            n271 = local read "Time_out"() -> (w854:bool)
            n272 = Wait (ms)(milliseconds to wait=u32 10) -> ()  [unwired: 1 out]
            n273 = Not(x=w854) -> (.not. x?=w853:bool)
            n274 = Not(x=w850) -> (.not. x?=w848:bool)
            n275 = Not(x=w844) -> (.not. x?=w845:bool)
            n276 = And(x=w853, y=w852) -> (x .and. y?=w847:bool)
            n277 = And(x=w849, y=w848) -> (x .and. y?=w843:bool)
            n278 = local read "Time_out"() -> (w851:bool)
            n279 = And(x=w842, y=w845) -> (x .and. y?=w841:bool)
            n280 = Or(x=w847, y=w843) -> (x .or. y?=w840:bool)
            n281 = Or(x=w840, y=w841) -> (x .or. y?=w839:bool)
            n282 = case shown="True" w839 {
              tunnel: w851 -> [w856 _]
              frame False {
                n283 = case shown="False" w856 {
                  frame False {
                    n284 = local read "ISI start time"() -> (w859:dbl)
                    n285 = local read "Time"() -> (w858:dbl)
                    n286 = Subtract(x=w858, y=w859) -> (x-y=w857:dbl)
                    n287 = shared-variable "My Computer\\michelle_library.lvlib\\ISI"(w857) -> ()  [unwired: 1 in, 1 out]
                    n288 = local write "ISI"(w857) -> ()
                  }
                  frame True {
                    n289 = local read "Time"() -> (w864:dbl)
                    n290 = Subtract(x=w864, y=0.11) -> (x-y=w861:dbl)
                    n291 = local write "ISI start time"(w861) -> ()
                    n292 = local read "Time"() -> (w862:dbl)
                    n293 = Subtract(x=w862, y=w861) -> (x-y=w860:dbl)
                    n294 = shared-variable "My Computer\\michelle_library.lvlib\\ISI"(w860) -> ()  [unwired: 1 in, 1 out]
                    n295 = local write "ISI"(w860) -> ()
                  }
                }
              }
              frame True {
                n296 = local read "Time"() -> (w869:dbl)
                n297 = Subtract(x=w869, y=0.11) -> (x-y=w866:dbl)
                "ISI start time" <- w866
                n298 = local read "Time"() -> (w867:dbl)
                n299 = Subtract(x=w867, y=w866) -> (x-y=w865:dbl)
                "ISI" <- w865
                n300 = shared-variable "My Computer\\michelle_library.lvlib\\ISI"(w865) -> ()  [unwired: 1 in, 1 out]
              }
            }
            n301 = local read "Stop"() -> (w855:bool)
          }
          n302 = while {
            stop <- w744 stop-if-true
            n303 = local read "Active Trial"() -> (w743:bool)
            n304 = case shown="True" w743 {
              frame False {
              }
              frame True {
                n305 = local write "Time_out"(FALSE) -> ()
                n306 = shared-variable "My Computer\\michelle_library.lvlib\\Timeout"(FALSE) -> ()  [unwired: 1 in, 1 out]
              }
            }
            n307 = Wait (ms)(milliseconds to wait=5) -> ()  [unwired: 1 out]
            n308 = shared-variable "My Computer\\michelle_library.lvlib\\Stop"() -> (w744:bool)  [unwired: 1 in, 1 out]
          }
          n309 = while {
            stop <- w765 stop-if-true
            n310 = shared-variable "My Computer\\michelle_library.lvlib\\Trial"() -> (w755:u32)  [unwired: 1 in, 1 out]
            n311 = Wait (ms)(milliseconds to wait=u32 10) -> ()  [unwired: 1 out]
            n312 = local read "Timings"() -> (w757:dbl[])
            n313 = local read "Time since lick"() -> (w764:dbl)
            n314 = Decrement(x=w755) -> (x-1=w754:u32)
            n315 = Index Array(array=w757, index=w754) -> (element=w756:dbl)
            n316 = Less?(x=w764, y=w756) -> (x < y?=w763:bool)
            n317 = shared-variable "My Computer\\michelle_library.lvlib\\Display"() -> (w760:bool)  [unwired: 1 in, 1 out]
            n318 = local read "ConsumptionGo"() -> (w752:bool)
            n319 = local read "Lick"() -> (w762:bool)
            n320 = And(x=w762, y=w763) -> (x .and. y?=w758:bool)
            n321 = Not(x=w760) -> (.not. x?=w759:bool)
            n322 = local read "Active Trial"() -> (w747:bool)
            n323 = And(x=w759, y=w758) -> (x .and. y?=w751:bool)
            n324 = Not(x=w752) -> (.not. x?=w753:bool)
            n325 = And(x=w751, y=w753) -> (x .and. y?=w749:bool)
            n326 = Not(x=w747) -> (.not. x?=w750:bool)
            n327 = And(x=w749, y=w750) -> (x .and. y?=w748:bool)
            n328 = case shown="True" w748 {
              frame False {
              }
              frame True {
                n329 = flat-sequence {
                  frame #0 {
                    w766 = TRUE
                    n330 = local read "TimeOutDuration"() -> (w767:i32)
                    n331 = xnode "DisplayOn 3"("C/DIO3 (DIO3)"=w766) -> ()  [unwired: 1 in, 1 out]
                    n332 = shared-variable "My Computer\\michelle_library.lvlib\\Timeout"(w766) -> ()  [unwired: 1 in, 1 out]
                    n333 = Wait (ms)(milliseconds to wait=w767) -> ()  [unwired: 1 out]
                    "Time_out" <- w766
                  }
                  frame #1 {
                    w803 = FALSE ("Timeout")
                    n334 = xnode "DisplayOn 4"("C/DIO3 (DIO3)"=w803) -> ()  [unwired: 1 in, 1 out]
                    n335 = local write "Time_out"(w803) -> ()
                    n336 = shared-variable "My Computer\\michelle_library.lvlib\\Timeout"(w803) -> ()  [unwired: 1 in, 1 out]
                  }
                }
              }
            }
            n337 = local read "Stop"() -> (w765:bool)
          }
          n338 = while {
            shift-right: [w916] -> _
            shift-left: _ -> [w915]
            shift-right: [w908] -> _
            shift-left: _ -> [w909]
            stop <- w918 stop-if-true
            n339 = local read "Active Trial"() -> (w913:bool)
            n340 = Wait (ms)(milliseconds to wait=u32 10) -> ()  [unwired: 1 out]
            n341 = local read "Lick"() -> (w914:bool)
            n342 = And(x=w913, y=w914) -> (x .and. y?=w912:bool)
            n343 = Or(x="Give reward", y=w912) -> (x .or. y?=w911:bool)
            n344 = case shown="True" w911 {
              tunnel: [w920 w927] -> w916
              tunnel: w915 -> [w920 w926]
              tunnel: w909 -> [w919 w924]
              tunnel: [w919 w923] -> w908
              frame False {
              }
              frame True {
                n345 = flat-sequence {
                  tunnel: w924 -> [w933]
                  tunnel: [w930] -> w921
                  tunnel: [w989] -> w922
                  tunnel: w921 -> [w987]
                  tunnel: [w1033] -> w923
                  tunnel: w922 -> [w1033]
                  frame #0 {
                    w948 = TRUE ("C/DIO0 (DIO0)")
                    n346 = Get Date/Time In Seconds() -> (seconds since 1Jan1904=w937:timestamp)
                    n347 = local write "Time_out"(FALSE) -> ()
                    n348 = shared-variable "My Computer\\michelle_library.lvlib\\Timeout"(FALSE) -> ()  [unwired: 1 in, 1 out]
                    n349 = local write "GoAhead"(FALSE) -> ()
                    n350 = Wait (ms)(milliseconds to wait=u32 100) -> ()  [unwired: 1 out]
                    n351 = local read "TestTime"() -> (w931:dbl)
                    n352 = shared-variable "My Computer\\michelle_library.lvlib\\Trial"() -> (w947:u32)  [unwired: 1 in, 1 out]
                    n353 = shared-variable "My Computer\\michelle_library.lvlib\\GlobalReward"() -> (w939:dbl)  [unwired: 1 in, 1 out]
                    n354 = To Double Precision Float(number=w937) -> (double precision float=w936:dbl)
                    n355 = shared-variable "My Computer\\michelle_library.lvlib\\GlobalTime"() -> (w929:dbl)  [unwired: 1 in, 1 out]
                    n356 = local read "Rewarded trials"() -> (w945:dbl[])
                    n357 = Subtract(x=w936, y=w931) -> (x-y=w935:dbl)
                    n358 = xnode "Reward 3"("C/DIO0 (DIO0)"=w948) -> ()  [unwired: 1 in, 1 out]
                    n359 = Decrement(x=w947) -> (x-1=w946:u32)
                    n360 = shared-variable "My Computer\\michelle_library.lvlib\\Frame_clock"() -> (w928:u32)  [unwired: 1 in, 1 out]
                    n361 = Increment(x=w939) -> (x+1=w938:dbl)
                    n362 = Replace Array Subset(array=w945, new element=1.0 ("new element/subarray"), index=w946) -> (w943:dbl[])
                    n363 = Build Array(551, w935, w929, w928) -> (w934:T1)
                    n364 = local write "Rewarded trials"(w943) -> ()
                    n365 = shared-variable "My Computer\\michelle_library.lvlib\\GlobalReward"(w938) -> ()  [unwired: 1 in, 1 out]
                    n366 = Build Array (concatenate) ("Build Matrix")(w933, w934) -> (w930:T1)
                    n367 = local write "RewTS"(w930) -> ()
                    "Reward" <- w948
                    "Watch_Display" <- w948
                  }
                  frame #1 {
                    w997 = FALSE ("C/DIO0 (DIO0)")
                    n368 = Get Date/Time In Seconds() -> (seconds since 1Jan1904=w994:timestamp)
                    n369 = local read "TestTime"() -> (w988:dbl)
                    n370 = local write "Give reward"(FALSE ("Give reward")) -> ()
                    n371 = Wait (ms)(milliseconds to wait=u32 20) -> ()  [unwired: 1 out]
                    n372 = shared-variable "My Computer\\michelle_library.lvlib\\GlobalTime"() -> (w986:dbl)  [unwired: 1 in, 1 out]
                    n373 = To Double Precision Float(number=w994) -> (double precision float=w993:dbl)
                    n374 = xnode "Reward 4"("C/DIO0 (DIO0)"=w997) -> ()  [unwired: 1 in, 1 out]
                    n375 = local write "Reward"(w997) -> ()
                    n376 = Subtract(x=w993, y=w988) -> (x-y=w992:dbl)
                    n377 = shared-variable "My Computer\\michelle_library.lvlib\\Frame_clock"() -> (w985:u32)  [unwired: 1 in, 1 out]
                    n378 = Build Array(552, w992, w986, w985) -> (w990:T1)
                    n379 = Build Array (concatenate) ("Build Matrix")(w987, w990) -> (w989:T1)
                    n380 = local write "RewTS"(w989) -> ()
                  }
                  frame #2 {
                    n381 = Wait (ms)(milliseconds to wait=u32 50) -> ()  [unwired: 1 out]
                  }
                }
                n382 = Increment(x=w926) -> (x+1=w927:u16)
                "Rewards" <- w927
                n383 = local write "Active Trial"(FALSE ("Active Trial")) -> ()
              }
            }
            n384 = local read "Stop"() -> (w918:bool)
          }
          n385 = while {
            stop <- w883 stop-if-true
            n386 = shared-variable "My Computer\\michelle_library.lvlib\\Trial"() -> (w879:u32)  [unwired: 1 in, 1 out]
            n387 = shared-variable "My Computer\\michelle_library.lvlib\\Trial"() -> (w875:u32)  [unwired: 1 in, 1 out]
            n388 = Wait (ms)(milliseconds to wait=u32 10) -> ()  [unwired: 1 out]
            n389 = local read "Rewarded trials"() -> (w876:dbl[])
            n390 = local read "Reward_mat"() -> (w878:dbl[])
            n391 = Decrement(x=w879) -> (x-1=w880:u32)
            n392 = Decrement(x=w875) -> (x-1=w874:u32)
            n393 = Index Array(array=w878, index=w880) -> (element=w881:dbl)
            n394 = Index Array(array=w876, index=w874) -> (element=w873:dbl)
            n395 = Equal To 0?(x=w873) -> (x = 0?=w872:bool)
            n396 = Equal?(x=w881, y=1.0) -> (x = y?=w871:bool)
            n397 = And(x=w871, y=w872) -> (x .and. y?=w870:bool)
            n398 = case shown="True" w870 {
              frame False {
                n399 = local write "Active Trial"(FALSE ("Active_trial")) -> ()
              }
              frame True {
                n400 = shared-variable "My Computer\\michelle_library.lvlib\\Trial"() -> (w886:u32)  [unwired: 1 in, 1 out]
                n401 = local read "Stim_ID"() -> (w888:dbl[])
                n402 = Decrement(x=w886) -> (x-1=w887:u32)
                n403 = Index Array(array=w888, index=w887) -> (element=w885:dbl)
                n404 = case shown="1, Default" w885 {
                  frame 1, Default {
                    n405 = shared-variable "My Computer\\michelle_library.lvlib\\ISI_Time"() -> (w894:dbl)  [unwired: 1 in, 1 out]
                    n406 = local read "ActiveTime"() -> (w889:dbl)
                    n407 = Less?(x=w894, y=w889) -> (x < y?=w892:bool)
                    n408 = Greater?(x=w894, y=0.1) -> (0:w891:bool)
                    n409 = And(x=w892, y=w891) -> (x .and. y?=w890:bool)
                    n410 = case shown="True" w890 {
                      frame False {
                        n411 = local write "Active Trial"(FALSE ("Active Trial")) -> ()
                      }
                      frame True {
                        n412 = local read "Time"() -> (w898:dbl)
                        n413 = local write "Active Trial"(TRUE ("Active Trial")) -> ()
                        n414 = Add(x=w898, y=-0.11) -> (x+y=w896:dbl)
                        n415 = local write "Time of last lick"(w896) -> ()
                      }
                    }
                  }
                  frame 2 {
                    n416 = shared-variable "My Computer\\michelle_library.lvlib\\ISI_Time"() -> (w904:dbl)  [unwired: 1 in, 1 out]
                    n417 = local read "ActiveTime"() -> (w900:dbl)
                    n418 = Less?(x=w904, y=w900) -> (x < y?=w902:bool)
                    n419 = Greater?(x=w904, y=0.1) -> (0:w903:bool)
                    n420 = And(x=w903, y=w902) -> (x .and. y?=w901:bool)
                    n421 = case shown="True" w901 {
                      frame False {
                        n422 = local write "Active Trial"(FALSE ("Active Trial")) -> ()
                      }
                      frame True {
                        "Active Trial" <- TRUE ("Active Trial")
                      }
                    }
                  }
                }
              }
            }
            n423 = local read "Stop"() -> (w883:bool)
          }
        }
      }
      n424 = while {
        shift-right: [w346] -> _
        shift-left: _ -> [w341]
        stop <- w345 stop-if-true
        n425 = xnode "PhotoDiode"() -> ("C/AI0 (AI0)"=w342:dbl)  [unwired: 1 in, 1 out]
        "Light" <- w342
        n426 = Wait (ms)(milliseconds to wait=u32 10) -> ()  [unwired: 1 out]
        n427 = Greater?(x=w342, y=0.5) -> (0:→"LightOn":bool)
        n428 = Build Array (concatenate)(w341, w342) -> (w346:dbl[])
        "Lightplot" <- w346
        "LightArray" <- w346
        n429 = local read "Stop"() -> (w345:bool)
      }
      n430 = flat-sequence {
        frame #0 {
          n431 = xnode "Encoder 4"("Reset Counter"=TRUE) -> ()  [unwired: 1 in, 4 out]
        }
        frame #1 {
          n432 = while {
            shift-right: [w438] -> _
            shift-left: _ -> [w439]
            stop <- w443 stop-if-true
            n433 = local read "GetVidFrame"() -> (w433:i32)
            n434 = local read "VidFrameClock"() -> (w437:i32)
            n435 = Equal?(x=w437, y=1) -> (x = y?=w436:bool)
            n436 = Equal?(x=w433, y=1) -> (x = y?=w432:bool)
            n437 = And(x=w436, y=w432) -> (x .and. y?=w435:bool)
            n438 = case shown="True" w435 {
              tunnel: w439 -> [w447 w450]
              tunnel: [w447 w449] -> w438
              frame False {
              }
              frame True {
                n439 = local read "TestTime"() -> (w456:dbl)
                n440 = shared-variable "My Computer\\michelle_library.lvlib\\GlobalTime"() -> (w453:dbl)  [unwired: 1 in, 1 out]
                n441 = Get Date/Time In Seconds() -> (seconds since 1Jan1904=w458:timestamp)
                n442 = shared-variable "My Computer\\michelle_library.lvlib\\Frame_clock"() -> (w454:u32)  [unwired: 1 in, 1 out]
                n443 = To Double Precision Float(number=w458) -> (double precision float=w457:dbl)
                n444 = Subtract(x=w457, y=w456) -> (x-y=w455:dbl)
                n445 = Build Array(881, w455, w453, w454) -> (w452:T1)
                n446 = Build Array (concatenate) ("Build Matrix")(w450, w452) -> (w449:T1)
                n447 = local write "GetVidFrame"(0) -> ()
                n448 = local write "VidTS"(w449) -> ()
              }
            }
            n449 = xnode "Encoder 3"() -> ("Counter Value"=w445:i32)  [unwired: 2 in, 3 out]
            n450 = Multiply(x=w445, y=-1) -> (x*y=w442:i32)
            "VidFrameClock" <- w442
            n451 = Equal?(x=w442, y=720000) -> (x = y?=w443:bool)
            n452 = shared-variable "My Computer\\michelle_library.lvlib\\VidFrameClock1"(w442) -> ()  [unwired: 1 in, 1 out]
            n453 = local write "Stop"(w443) -> ()
            n454 = Wait (ms)(milliseconds to wait=u32 1) -> ()  [unwired: 1 out]
          }
        }
        frame #2 {
          n455 = local read "Stop"() -> (w505:bool)
          n456 = shared-variable "My Computer\\michelle_library.lvlib\\Stop"(w505) -> ()  [unwired: 1 in, 1 out]
        }
      }
    }
  }
